vi "图像平移旋转.vi"() -> ()   [LabVIEW 2018]
uses:
  <vilib>/vision/NI_Vision_Development_Module.lvlib
panel:
  out "error out":errorcluster
  out "Image 3":T1(plugin-control)
  out "Image 2":T1(plugin-control)
  out "Image":T1(plugin-control)
  in  "路径":path
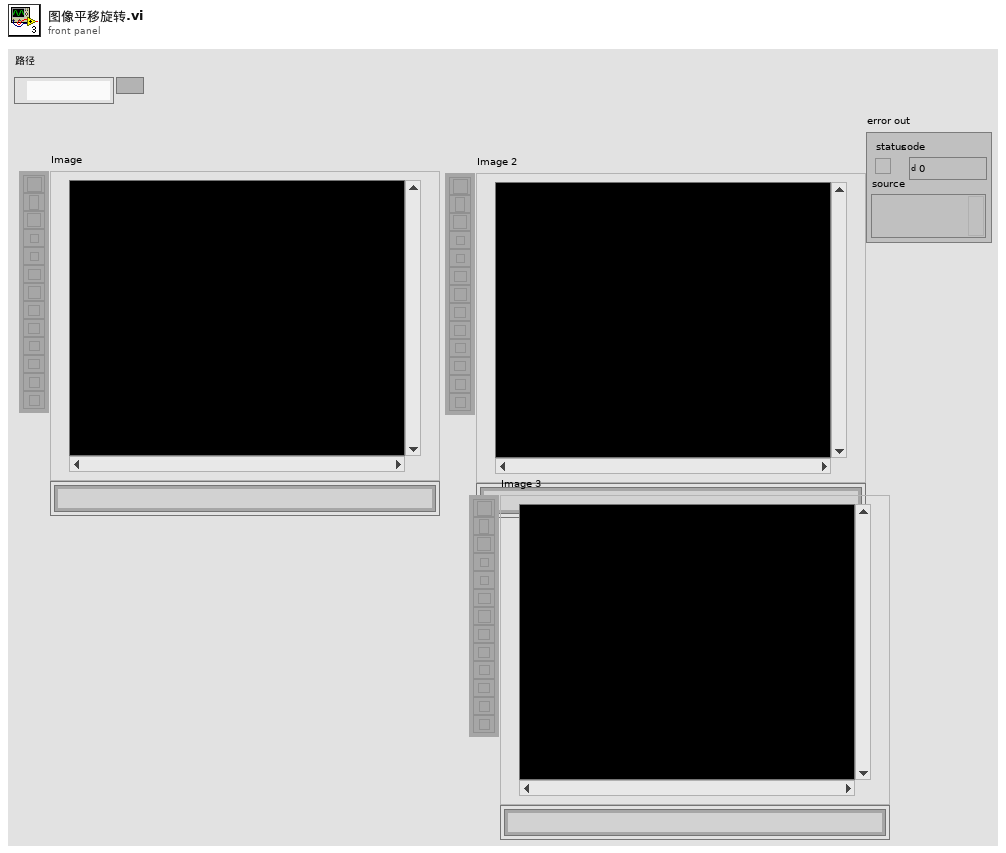
[diagram p1: front panel]
types:
  T1 = typedef "IMAQ Image.ctl" = refnum<image>
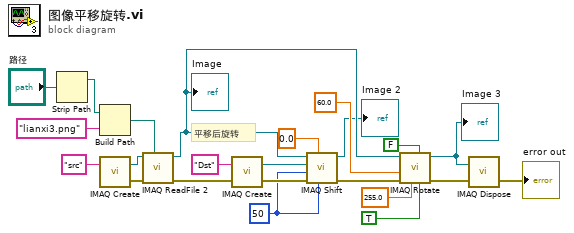
[diagram p0: block diagram]
diagram:
  w12 = 50 ("XOffset")
  # "平移后旋转"
  n1 = Strip Path(path="路径") -> (stripped path=w22:path)  [unwired: 1 out]
  n2 = Build Path(base path=w22, name or relative path="lianxi3.png" ("名称或相对路径")) -> (appended path=w18:path)
  n3 = call "IMAQ Create"("Image Name"="src") -> ("New Image"=w20:T1, "error out"=w19:errorcluster)  [unwired: 4 in]
  n4 = call "IMAQ ReadFile 2"("File Path"=w18, "error in (no error)"=w19, "Image"=w20) -> ("error out"=w14:errorcluster, "Image Out"=w6:T1)  [unwired: 4 in, 3 out]
  "Image" <- w6
  n5 = call "IMAQ Create"("Image Name"="Dst", "error in (no error)"=w14) -> ("New Image"=w16:T1, "error out"=w15:errorcluster)  [unwired: 3 in]
  n6 = call "IMAQ Shift"("YOffset"=w12, "Replace Value"=sgl 0.0, "error in (no error)"=w15, "XOffset"=w12, "Image Dst"=w16, "Image Src"=w6) -> ("error out"=w10:errorcluster, "Image Dst Out"=→"Image 2":T1)  [unwired: 4 in]
  n7 = call "IMAQ Rotate"("Use Bilinear Interpolation"=TRUE, "Maintain Size"=FALSE, "Replace Value"=sgl 255.0, "error in (no error)"=w10, "Angle (degrees)"=sgl 60.0, "Image Src"=w6) -> ("error out"=w3:errorcluster, "Image Dst Out"=w4:T1)  [unwired: 4 in]
  "Image 3" <- w4
  n8 = call "IMAQ Dispose"("Image"=w4, "error in (no error)"=w3) -> ("error out"=→"error out":errorcluster)  [unwired: 4 in]
